vi "ShooterTEST.vi"(5 "WinchCaseIn":dbl, 8 "OutGearPos":dbl=2.1, 9 "InGearPos":dbl=1.5, 10 "Pot":dbl, 11 "Fire":bool) -> (0 "There?":bool, 1 "WinchCase":i32, 3 "Power":dbl)   [LabVIEW 2013]
panel:
  out "Index":i32
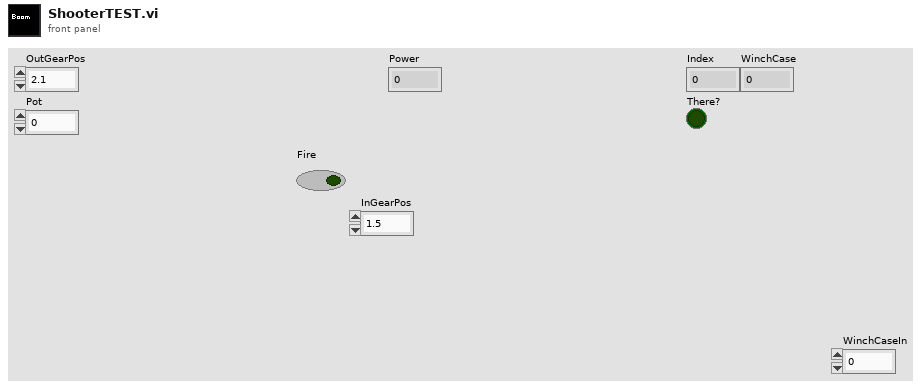
[diagram p1: front panel]
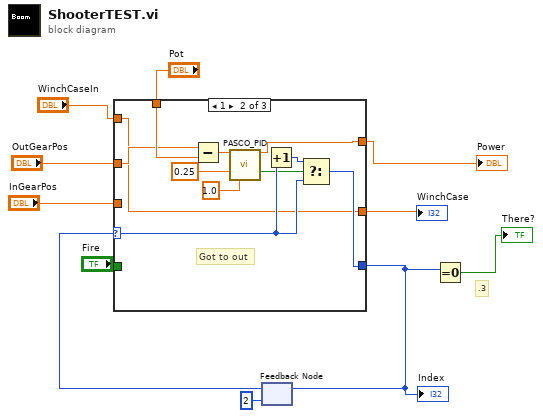
[diagram p0: block diagram]
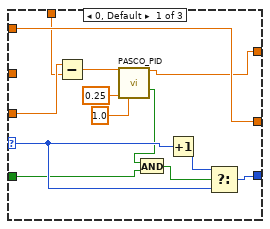
[diagram p2: hidden frame]
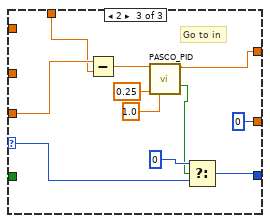
[diagram p3: hidden frame]
diagram:
  # ".3"
  n1 = feedback #1(2 ("Numeric")) -> (w9:i32)
  n2 = case shown="1" w9 {
    selector: w9 -> [w22 w33 w44]
    tunnel: [w14 w32 w37] -> w1
    tunnel: "Fire" -> [w15 _ _]
    tunnel: [w24 w35 w46] -> w6
    tunnel: "OutGearPos" -> [_ w28 _]
    tunnel: "InGearPos" -> [w19 _ w42]
    tunnel: "Pot" -> [w18 w29 w41]
    tunnel: [w21 w27 0 ("WinchCase")] -> w3
    tunnel: "WinchCaseIn" -> [w21 w27 _]
    frame 0, Default {
      n3 = Subtract(x=w19, y=w18) -> (x-y=w20:dbl)
      n4 = call "PASCO_PID.vi"("Delta"=w20, "Deadband"=0.25, "P Gain"=1.0) -> ("Output"=w14:dbl, "IsThere"=w16:bool)  [unwired: 11 in]
      n5 = And(x=w16, y=w15) -> (x .and. y?=w17:bool)
      n6 = Increment(x=w22) -> (x+1=w23:i32)
      n7 = Select(t=w23, s=w17, f=w22) -> (s? t:f=w24:i32)
    }
    frame 1 {
      # "Got to out"
      n8 = Subtract(x=w28, y=w29) -> (x-y=w30:dbl)
      n9 = call "PASCO_PID.vi"("Delta"=w30, "Deadband"=0.25, "P Gain"=1.0) -> ("Output"=w32:dbl, "IsThere"=w31:bool)  [unwired: 11 in]
      n10 = Increment(x=w33) -> (x+1=w34:i32)
      n11 = Select(t=w34, s=w31, f=w33) -> (s? t:f=w35:i32)
    }
    frame 2 {
      # "Go to in"
      n12 = Subtract(x=w42, y=w41) -> (x-y=w40:dbl)
      n13 = call "PASCO_PID.vi"("Delta"=w40, "Deadband"=0.25, "P Gain"=1.0) -> ("Output"=w37:dbl, "IsThere"=w43:bool)  [unwired: 11 in]
      n14 = Select(t=0, s=w43, f=w44) -> (s? t:f=w46:i32)
    }
  }
  "Power" <- w1
  "Index" <- w6
  "WinchCase" <- w3
  n15 = feedback-in #1(w6) -> ()
  n16 = Equal To 0?(x=w6) -> (x = 0?=→"There?":bool)
